vi "practica7transferencia.vi"() -> ()   [LabVIEW 2016]
panel:
  out "Distancia":dbl
  out "Angulo":dbl
  out "Plano de trabajo":picture
  in  "Reset":bool
  in  "stop":bool
  out "Motor Izquierda":dbl(slide) scale=-100.0..100.0
  out "Motor Derecha":dbl(slide) scale=-100.0..100.0
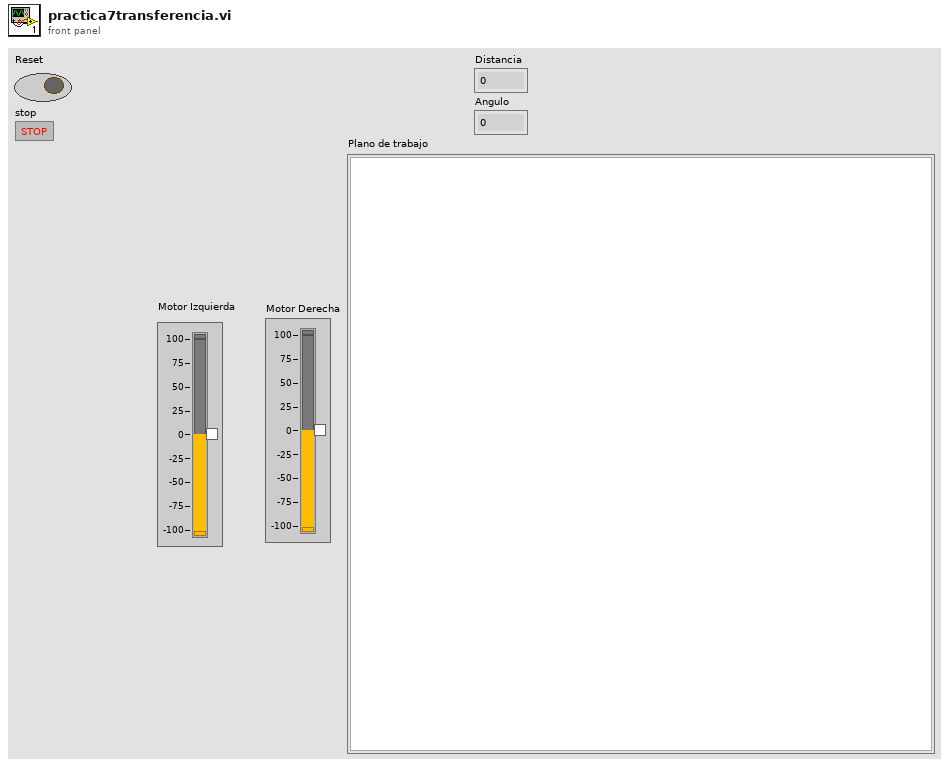
[diagram p1: front panel]
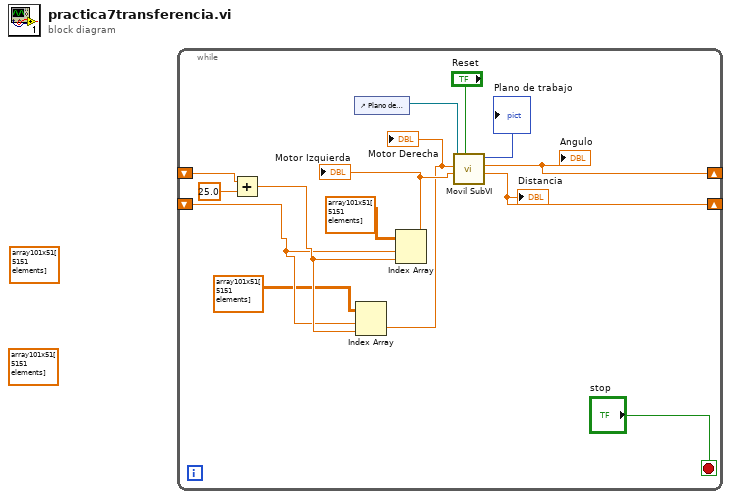
[diagram p0: block diagram]
diagram:
  (unwired) dbl[][] array101x51[5151 elements] ("izquierdo")
  (unwired) dbl[][] array101x51[5151 elements] ("derecho")
  n1 = while {
    shift-right: [w10] -> _
    shift-left: _ -> [w8]
    shift-right: [w9] -> _
    shift-left: _ -> [w5]
    stop <- "stop" stop-if-true
    n2 = Add(x=w8, y=25.0) -> (x+y=w6:dbl)
    n3 = control-ref of="Plano de trabajo"() -> (w13:refnum<vi>)
    n4 = Index Array(array=dbl[][] array101x51[5151 elements] ("Waveform Chart 2"), index (row)=w5, index (col)=w6) -> (element=w1:dbl)
    "Motor Derecha" <- w1
    n5 = Index Array(array=dbl[][] array101x51[5151 elements] ("Waveform Chart"), index (row)=w5, index (col)=w6) -> (element=w2:dbl)
    "Motor Izquierda" <- w2
    n6 = call "Movil SubVI.vi"("Reset"="Reset", "Motor Izquierda"=w2, "Motor Derecha"=w1, "Ref Plano"=w13) -> ("Distancia"=w9:dbl, "Angulo"=w10:dbl, "Plano de trabajo"=→"Plano de trabajo":picture)  [unwired: 3 in, 2 out]
    "Distancia" <- w9
    "Angulo" <- w10
  }
